vi "Get Data.vi"(8 "error in (no error)":errorcluster, 11 "MCListbox with Checkboxes in":refnum<class "MCListbox with Checkboxes.lvclass">) -> (0 "error out":errorcluster, 1 "Check Data":bool[](array[boolean]), 2 "Cell Data":string[][](array[string]), 3 "MCListbox with Checkboxes out":refnum<class "MCListbox with Checkboxes.lvclass">)   [LabVIEW 2016, in "MCListbox with Checkboxes.lvclass"]
uses:
  MCListbox with Checkboxes.lvclass
  MCListbox with Checkboxes.lvclass/MCListbox with Checkboxes.ctl
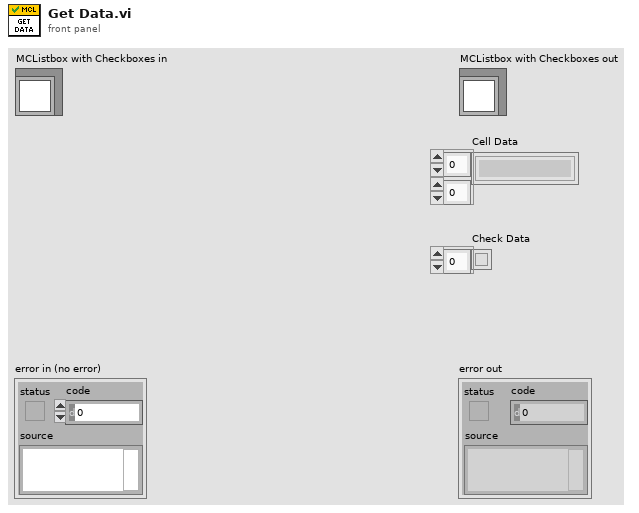
[diagram p1: front panel]
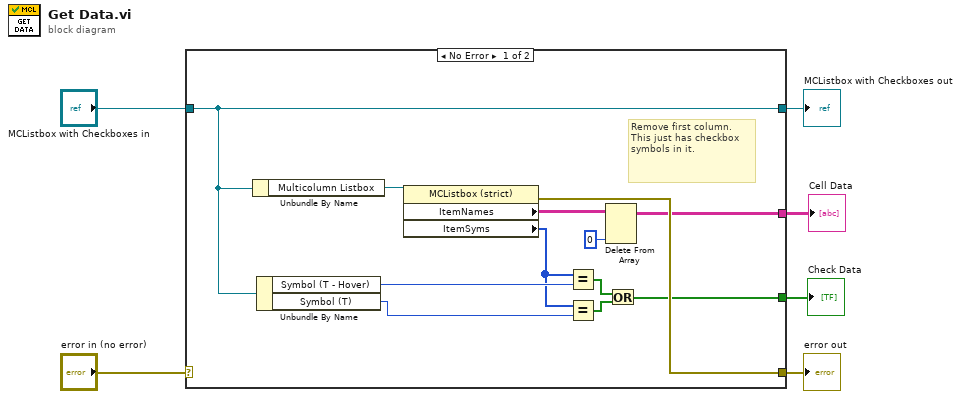
[diagram p0: block diagram]
diagram:
  n1 = case shown="No Error" "error in (no error)" {
    selector: "error in (no error)" -> [_ w20]
    tunnel: [w18 w20] -> w5
    tunnel: [w16 w19] -> w3
    tunnel: "MCListbox with Checkboxes in" -> [w16 w19]
    tunnel: [w10 _] -> w2
    tunnel: [w7 _] -> w1
    frame No Error {
      # "Remove first column. This just has checkbox symbols in it."
      n2 = Unbundle By Name(w16) -> ("Multicolumn Listbox"=w17:refnum<vi>)
      n3 = Unbundle By Name(w16) -> ("Symbol (T - Hover)"=w15:i32, "Symbol (T)"=w13:i32)
      n4 = property class="MCListbox (strict)"(reference=w17) -> (error out=w18:errorcluster, "ItemNames"=w9:string[][], "ItemSyms"=w14:i32[])  [unwired: 1 in, 1 out]
      n5 = Equal?(x=w14, y=w15) -> (x = y?=w12:bool[])
      n6 = Equal?(x=w14, y=w13) -> (x = y?=w11:bool[])
      n7 = Delete From Array(array=w9, index (col)=0 ("disabled index (col)")) -> (array with subset deleted=w7:string[][])  [unwired: 2 in, 1 out]
      n8 = Or(x=w12, y=w11) -> (x .or. y?=w10:bool[])
    }
    frame Error {
    }
  }
  "error out" <- w5
  "MCListbox with Checkboxes out" <- w3
  "Cell Data" <- w1
  "Check Data" <- w2
